vi "Update.vi"(8 "error in (no error)":errorcluster, 10 "Audio Block In":dbl[][](array[numeric]), 11 "Channel in":refnum<class "Channel.lvclass">) -> (0 "error out":errorcluster, 1 "Headphones Audio Block Out":dbl[][](array[numeric]), 2 "Master Audio Block Out":dbl[][](array[numeric]), 3 "Channel out":refnum<class "Channel.lvclass">)   [LabVIEW 2019, in "Channel.lvclass"]
uses:
  Channel.lvclass
  Channel.lvclass/Channel.ctl
  Packed Libraries/Globals.lvlibp/Constants.vi
  Packed Libraries/Globals.lvlibp
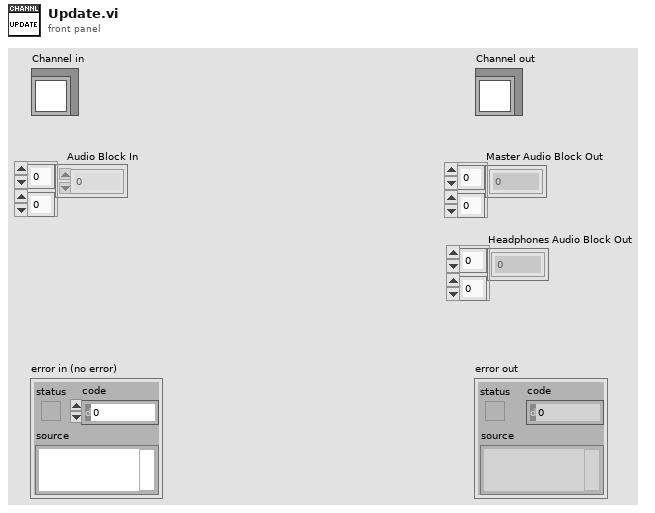
[diagram p1: front panel]
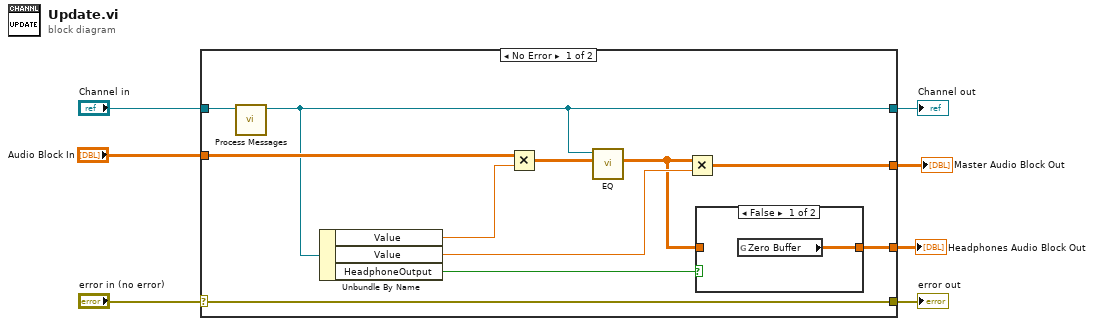
[diagram p0: block diagram]
diagram:
  n1 = case shown="No Error" "error in (no error)" {
    selector: "error in (no error)" -> [w18 w23]
    tunnel: [w18 w23] -> w6
    tunnel: [w9 w22] -> w4
    tunnel: "Channel in" -> [w8 w22]
    tunnel: [w15 w21] -> w3
    tunnel: "Audio Block In" -> [w11 w21]
    tunnel: [w13 w21] -> w1
    frame No Error {
      n2 = call "Process Messages.vi"("Channel in"=w8) -> ("Channel out"=w9:refnum<class "Channel.lvclass">)  [unwired: 9 in, 1 out]
      n3 = Unbundle By Name(w9) -> ("Value"=w17:dbl, "Value"=w16:dbl, "HeadphoneOutput"=w14:bool)
      n4 = Multiply(x=w11, y=w17) -> (x*y=w10:dbl[][])
      n5 = call "EQ.vi"("Audio Block In"=w10, "Channel in"=w9) -> ("Audio Block Out"=w12:dbl[][])  [unwired: 8 in, 1 out]
      n6 = Multiply(x=w12, y=w16) -> (x*y=w15:dbl[][])
      n7 = case shown="False" w14 {
        tunnel: [w19 w20] -> w13
        tunnel: w12 -> [_ w20]
        frame False {
          n8 = global read "Constants.vi" "Zero Buffer"() -> (w19:dbl[][])
        }
        frame True {
        }
      }
    }
    frame Error {
    }
  }
  "error out" <- w6
  "Channel out" <- w4
  "Master Audio Block Out" <- w3
  "Headphones Audio Block Out" <- w1
